vi "diviseur de tension.vi"() -> ()   [LabVIEW 2014]
panel:
  in  "Vin":dbl
  out "Vout":dbl
  in  "R2":dbl
  in  "R1":dbl
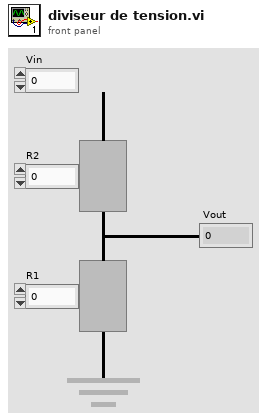
[diagram p1: front panel]
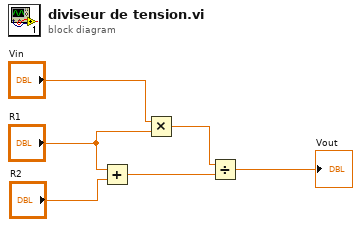
[diagram p0: block diagram]
diagram:
  n1 = Add(x="R1", y="R2") -> (x+y=w2:dbl)
  n2 = Multiply(x="Vin", y="R1") -> (x*y=w3:dbl)
  n3 = Divide(x=w3, y=w2) -> (x/y=→"Vout":dbl)
